vi "Configure Channel Location Offset.vi"(8 "error in (no error)":errorcluster, 9 "Channel Offset (0 meter)":dbl, 10 "Channel (1: Channel 1)":i32(ring)=1 items=["Channel 1"=1, "Channel 1.1"=11, "Channel 1.2"=12, "Channel 1.3"=13, "Channel 1.4"=14, "Channel 2"=2, "Channel 2.1"=21, "Channel 2.2"=22, "Channel 2.3"=23, "Channel 2.4"=24, "Channel 3"=3, "Channel 3.1"=31, "Channel 3.2"=32, "Channel 3.3"=33, "Channel 3.4"=34, "Channel 4"=4, "Channel 4.1"=41, "Channel 4.2"=42, "Channel 4.3"=43, "Channel 4.4"=44], 11 "VISA resource name":refnum<visa-resource-name>) -> (0 "error out":errorcluster, 3 "VISA resource name out":refnum<visa-resource-name>)   [LabVIEW 2015, in "Micron Optics sm130.lvlib"]
doc: "Configures the stored location calibration offset for the specified channel."
uses:
  Micron Optics sm130.lvlib
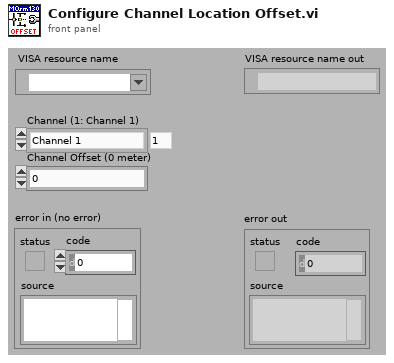
[diagram p1: front panel]
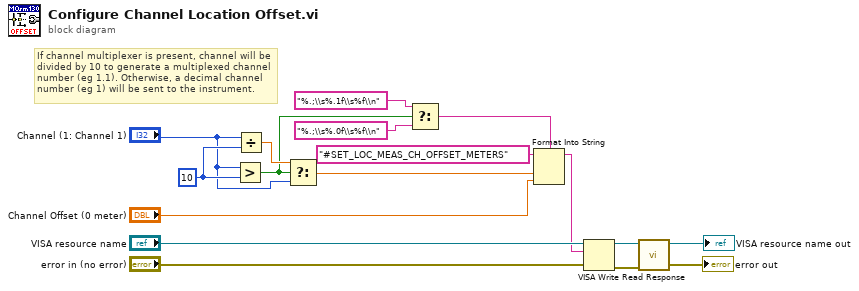
[diagram p0: block diagram]
diagram:
  w10 = 10 ("y")
  # "If channel multiplexer is present, channel will be divided by 10 to generate a multiplexed channel number (eg 1.1). Otherwise, a decimal channel number (eg 1) will be sent to the instrument."
  n1 = Greater?(x="Channel (1: Channel 1)", y=w10) -> (0:w9:bool)
  n2 = Divide(x="Channel (1: Channel 1)", y=w10) -> (x/y=w11:dbl)
  n3 = Select(t=w11, s=w9, f="Channel (1: Channel 1)") -> (s? t:f=w6:dbl)
  n4 = Select(t="%.;\\s%.1f\\s%f\\n" ("format string"), s=w9, f="%.;\\s%.0f\\s%f\\n" ("format string")) -> (s? t:f=w7:string)
  n5 = Format Into String(format string=w7, initial string="#SET_LOC_MEAS_CH_OFFSET_METERS", w6, "Channel Offset (0 meter)") -> (resulting string=w1:string)  [unwired: 1 in, 1 out]
  n6 = VISA Write(VISA resource name="VISA resource name", write buffer=w1, error in (no error)="error in (no error)") -> (VISA resource name out=w15:refnum<visa-resource-name>, error out=w14:errorcluster)  [unwired: 1 out]
  n7 = call "Read Response.vi"("error in (no error)"=w14, "VISA resource name"=w15) -> ("error out"=→"error out":errorcluster, "VISA resource name out"=→"VISA resource name out":refnum<visa-resource-name>)  [unwired: 7 in, 1 out]
